vi "AvgFuelArrayFix.vi"(11 "AvgFuelArrayin":dbl[][][](array[numeric])) -> (3 "AvgFuelArrayout":dbl[][][](array[numeric]))   [LabVIEW 2017]
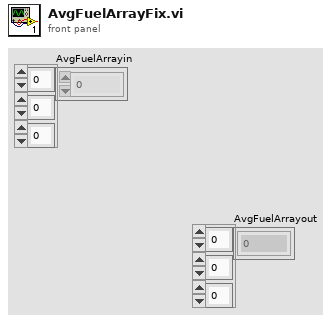
[diagram p1: front panel]
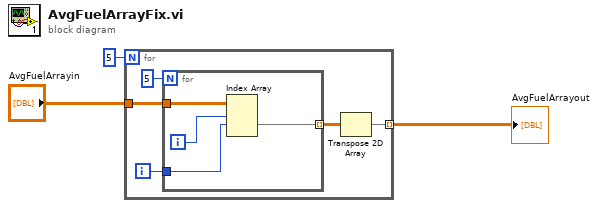
[diagram p0: block diagram]
diagram:
  n1 = for {
    N: 5 -> [_]
    tunnel: "AvgFuelArrayin" -> [w7]
    tunnel: [w4] -> w2 mode=indexing
    i -> [w6]
    n2 = for {
      N: 5 -> [_]
      tunnel: w7 -> [w11]
      tunnel: w6 -> [w10]
      tunnel: [w9] -> w5 mode=indexing
      i -> [w12]
      n3 = Index Array(array=w11, index (dim 0)=w12, index (dim 1)=w10) -> (element=w9:dbl[])  [unwired: 1 in]
    }
    n4 = Transpose 2D Array(2D array=w5) -> (transposed array=w4:dbl[][])
  }
  "AvgFuelArrayout" <- w2
